vi "Separa String.vi"(1 "TEXTO DE ENTRADA":string) -> (0 "VETOR DE SAIDA":dbl[](array[numeric]))   [LabVIEW 2018]
panel:
  out "Quantidade de Vírgulas":i32
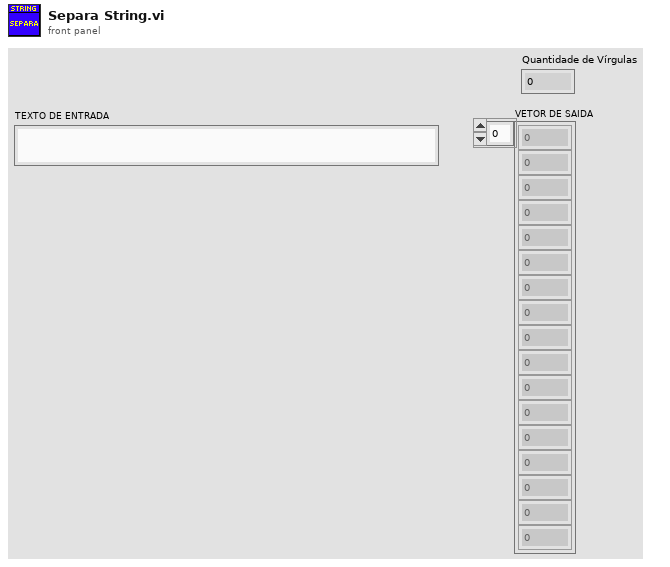
[diagram p1: front panel]
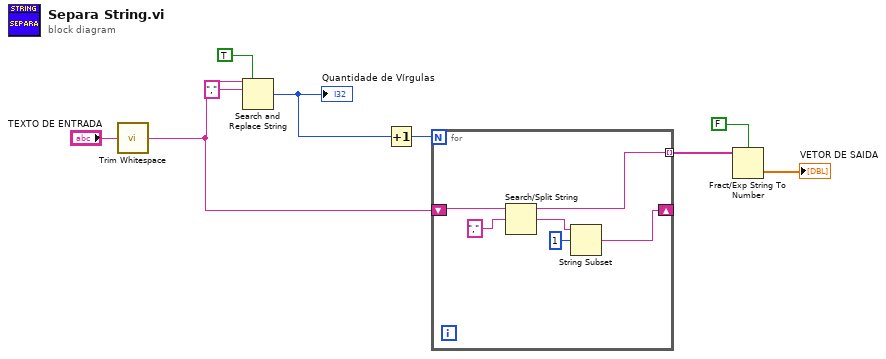
[diagram p0: block diagram]
diagram:
  n1 = call <vilib>:"Trim Whitespace.vi"("string"="TEXTO DE ENTRADA") -> ("trimmed string"=w5:string)  [unwired: 1 in]
  n2 = Search and Replace String(replace all?=TRUE ("replace all? (F)"), input string=w5, search string=",") -> (number of replacements=w1:i32)  [unwired: 5 in, 3 out]
  "Quantidade de Vírgulas" <- w1
  n3 = Increment(x=w1) -> (x+1=w2:i32)
  n4 = for {
    N: w2 -> [_]
    shift-right: [w11] -> _
    shift-left: w5 -> [w15]
    tunnel: [w10] -> w8 mode=indexing
    n5 = Search/Split String(string=w15, search string/char (-)=",") -> (substring before match=w10:string, match + rest of string=w13:string)  [unwired: 1 in, 1 out]
    n6 = String Subset(string=w13, offset (0)=1) -> (substring=w11:string)  [unwired: 1 in]
  }
  n7 = Fract/Exp String To Number(use system decimal point (T)=FALSE, string=w8) -> (number=→"VETOR DE SAIDA":dbl[])  [unwired: 2 in, 1 out]
